vi "main.vi"(8 "error in":errorcluster) -> (0 "error out":errorcluster)   [LabVIEW 2018, in "Vehicle Position Interface.lvlib"]
uses:
  Vehicle Position Interface.lvlib
  Common/Common.lvlib
  Common/vi/Stop All - Action.ctl
  ctl/Queue Actions.ctl
  ctl/Module State.ctl
  Error Handler/Error Handler/ctl/Module State.ctl
  Error Handler/Error Handler/Error Handler.lvlib
  Controller/Controller.lvlib
  Controller/ctl/Module State.ctl
  ctl/Vehicle Position.ctl
panel:
  in  "Vehicle Position":T1 scale=0.0..4.0
  # "[Covers: UI1]"
  # "Vehicle Position Simulation"
  # "[Covers: UI4]"
  # "[Covers: UI4A]"
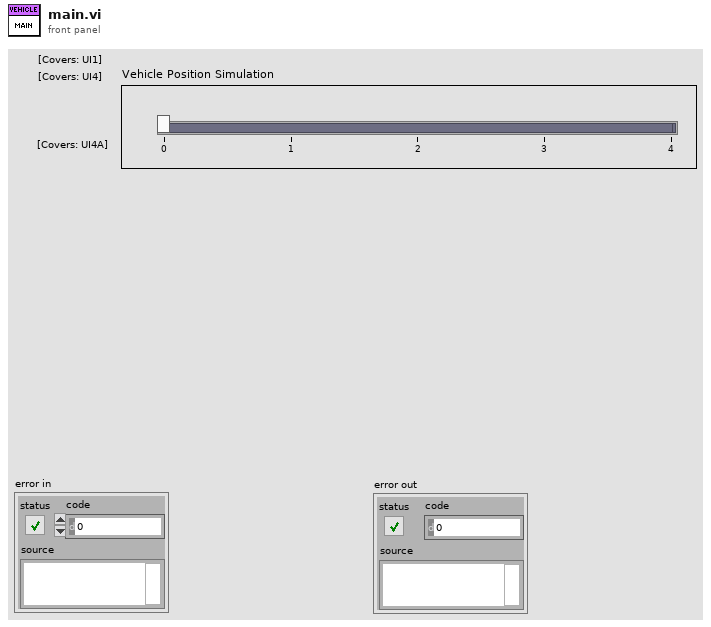
[diagram p1: front panel]
types:
  T1 = typedef "Vehicle Position Interface.lvlib/Vehicle Position.ctl" = dbl
  T2 = typedef "Vehicle Position Interface.lvlib/Module State.ctl" = enum16{"Init", "Idle", "Error", "Close", "Vehicle Position: Set", "Vehicle Position: Send to controller"}
  T3 = typedef "Vehicle Position Interface.lvlib/Queue Actions.ctl" = enum16{"Create", "Get", "Destroy"}
  T4 = typedef "Common.lvlib/Stop All - Action.ctl" = enum16{"Create", "Get", "Fire", "Destroy"}
  T5 = typedef "Controller.lvlib/Module State.ctl" = enum16{"Init", "Idle", "Error", "Close", "Wait for Start State", "Start State", "Wait For Vehicle Position", "Wash Step Execution", "Wash Step/Cycle Completion", "Wash Exit State", "Wash Abort/Terminate State", "Entry Console: Start button pressed", "Entry Console: Wash Steps buttons Pressed", "Vehicle Position: Slider Moved", "Check Timer"}
  T6 = typedef "Error Handler.lvlib/Module State.ctl" = enum16{"Init", "Idle", "Error", "Close", "Handle External Error", "Log Error"}
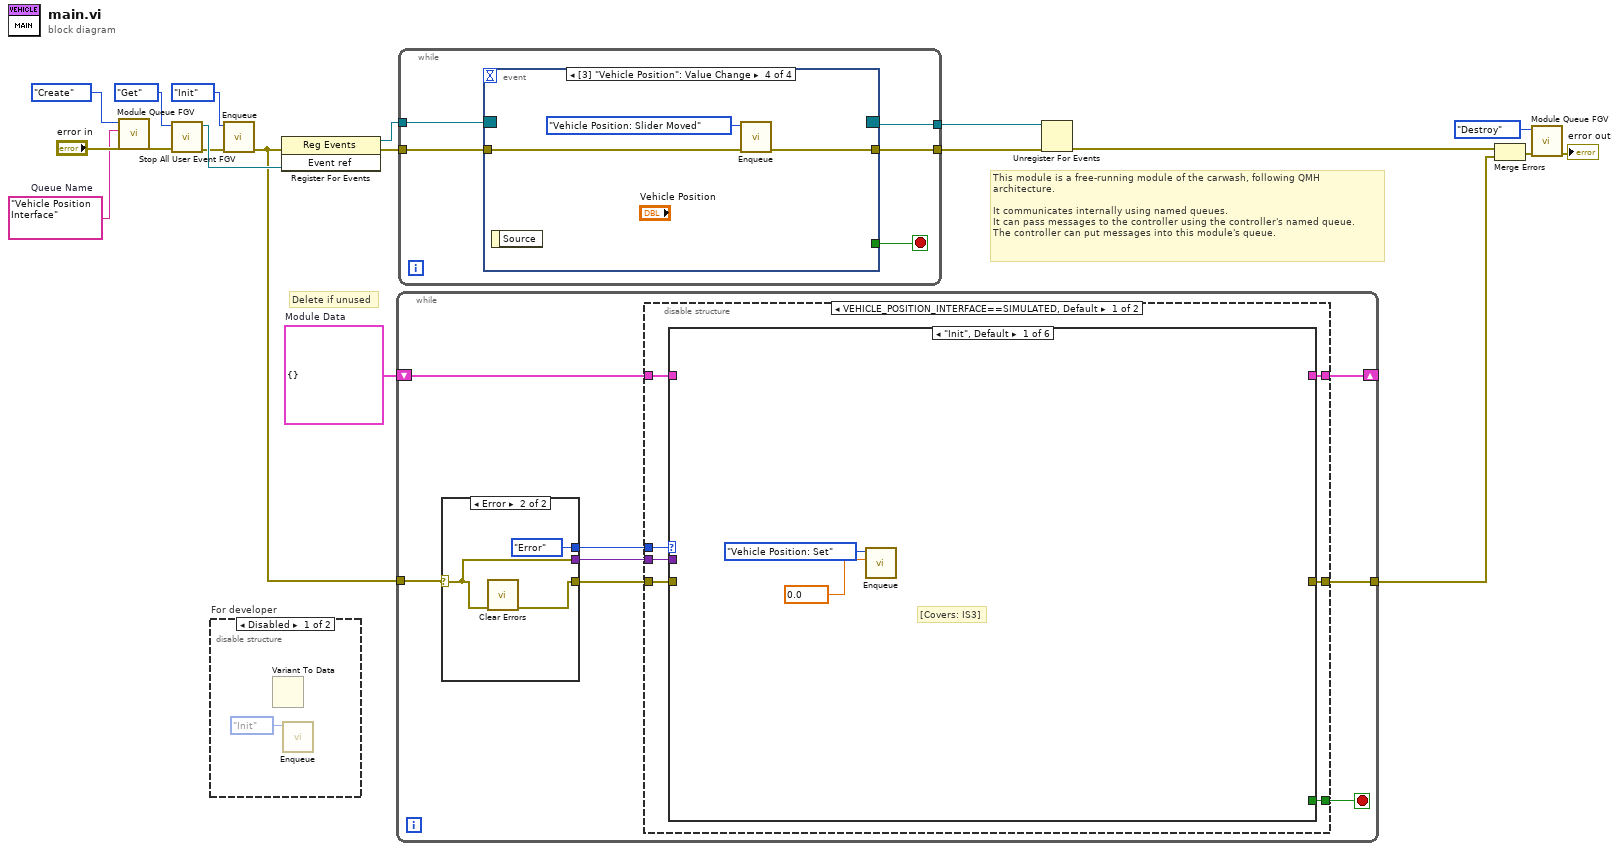
[diagram p0: block diagram]
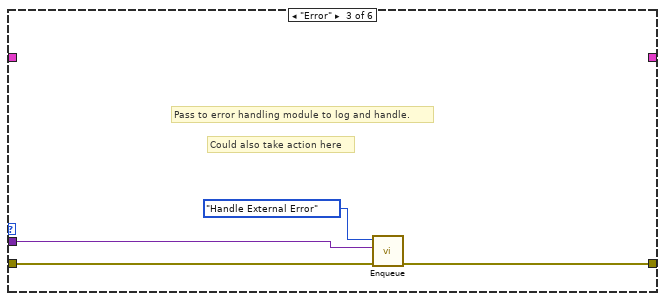
[diagram p4: hidden frame]
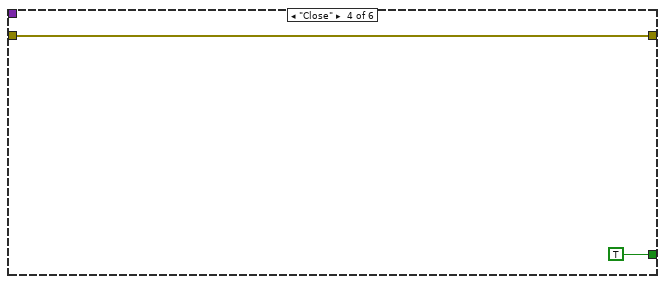
[diagram p5: hidden frame]
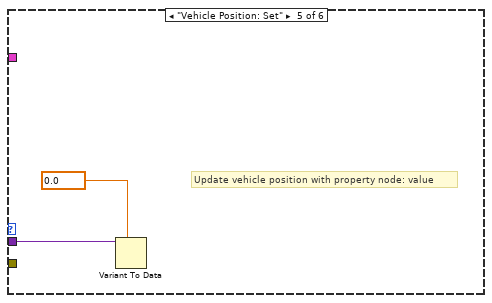
[diagram p6: hidden frame]
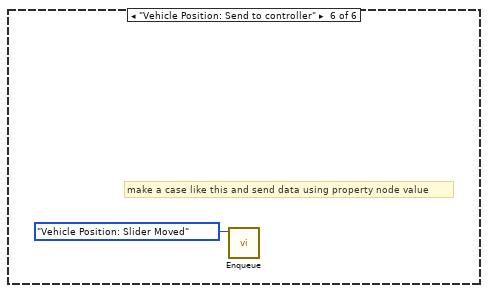
[diagram p7: hidden frame]
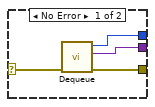
[diagram p9: hidden frame]
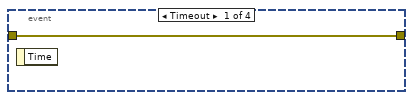
[diagram p10: hidden frame]
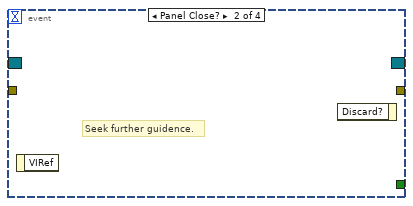
[diagram p11: hidden frame]
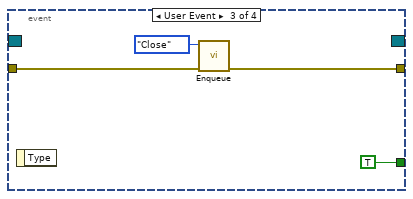
[diagram p12: hidden frame]
diagram:
  w1 = "Vehicle Position Interface"  # Queue Name
  w6 = cluster{} {}  # Module Data
  # "This module is a free-running module of the carwash, following QMH\narchitecture.\n\nIt communicates internally using named queues.\nIt can pass messages to the controller using the controller's named queue.\nThe controller can put messages into this module's queue."
  # "Delete if unused"
  n1 = call "Module Queue FGV.vi"("error in"="error in", "Queue Name"=w1, "Action"=Queue_Actions."Create") -> ("error out"=w16:errorcluster)  [unwired: 7 in, 1 out]
  n2 = call "Stop All User Event FGV.vi"("error in"=w16, "Action"=Stop_All_-_Action."Get") -> ("error out"=w15:errorcluster, "Event ref"=w18:refnum<user-event>)  [unwired: 8 in]
  n3 = disable-structure "For developer" shown="Disabled" {
    frame Disabled {
      n4 = Variant To Data() -> ()  [unwired: 3 in, 2 out]
      n5 = call "Enqueue.vi"("State"=Module_State."Init") -> ()  [unwired: 10 in, 1 out]
    }
    frame Enabled {
    }
  }
  n6 = call "Enqueue.vi"("error in"=w15, "State"=Module_State."Init") -> ("error out"=w7:errorcluster)  [unwired: 9 in]
  n7 = register-events(error in=w7, w18) -> (reference out=w13:refnum<event-registration>, error out=w11:errorcluster)  [unwired: 1 in]
  n8 = while {
    tunnel: w7 -> [w28]
    shift-right: [w23] -> _
    shift-left: w6 -> [w24]
    tunnel: [w21] -> w5
    stop <- w22 stop-if-true
    n9 = case shown="Error" w28 {
      selector: w28 -> [w51 w53]
      tunnel: [w50 w54] -> w25
      tunnel: [w49 w53] -> w26
      tunnel: [w48 Module_State."Error" ("State")] -> w27
      frame No Error {
        n10 = call "Dequeue.vi"("error in"=w51) -> ("error out"=w50:errorcluster, "Data"=w49:variant, "State"=w48:T2)  [unwired: 8 in]
      }
      frame Error {
        n11 = call <vilib>:"Clear Errors.vi"("error in (no error)"=w53) -> ("error out"=w54:errorcluster)  [unwired: 5 in, 1 out]
      }
    }
    n12 = disable-structure shown="VEHICLE_POSITION_INTERFACE==SIMULATED, Default" {
      disable-tunnel: w27 -> [w35 _]
      disable-tunnel: w26 -> [w34 _]
      disable-tunnel: w25 -> [w33 _]
      disable-tunnel: w24 -> [w32 _]
      disable-tunnel: [w31 _] -> w23
      disable-tunnel: [w30 _] -> w22
      disable-tunnel: [w29 _] -> w21
      frame condition #0 (active) {
        n13 = case shown="\"Init\", Default" w35 {
          tunnel: w34 -> [_ _ w40 _ w45 _]
          tunnel: w33 -> [_ _ w39 w43 _ _]
          tunnel: w32 -> [_ w38 _ _ _ _]
          tunnel: [_ w38 _ _ _ _] -> w31
          tunnel: [_ _ _ TRUE _ _] -> w30
          tunnel: [_ _ w41 w43 _ _] -> w29
          frame "Init", Default {
            w36 = 0.0 items=["Entry", "Station 1", "Station 2", "Station 3", "Exit"] ("Vehicle Position")
            # "[Covers: IS3]"
            n14 = call "Enqueue.vi"("Data"=w36, "State"=Module_State."Vehicle Position: Set") -> ()  [unwired: 9 in, 1 out]
          }
          frame "Idle" {
          }
          frame "Error" {
            # "Could also take action here"
            # "Pass to error handling module to log and handle."
            n15 = call "Enqueue.vi"("error in"=w39, "Data"=w40, "State"=Module_State."Handle External Error") -> ("error out"=w41:errorcluster)  [unwired: 8 in]
          }
          frame "Close" {
          }
          frame "Vehicle Position: Set" {
            w46 = 0.0 items=["Entry", "Station 1", "Station 2", "Station 3", "Exit"] ("Vehicle Position")
            # "Update vehicle position with property node: value"
            n16 = Variant To Data(type=w46, Variant=w45) -> ()  [unwired: 1 in, 2 out]
          }
          frame "Vehicle Position: Send to controller" {
            # "make a case like this and send data using property node value"
            n17 = call "Enqueue.vi"("State"=Module_State."Vehicle Position: Slider Moved") -> ()  [unwired: 10 in, 1 out]
          }
        }
      }
      frame condition #1 {
      }
    }
  }
  n18 = while {
    tunnel: w13 -> [w59]
    tunnel: [w58] -> w12
    tunnel: [w57] -> w10
    tunnel: w11 -> [w56]
    stop <- w55 stop-if-true
    n19 = event shown="[3] \"Vehicle Position\": Value Change" {
      selector: w59 -> [_ _ _ _]
      dyn-events: [_ _ _ _] -> w58
      timeout: _ -> [_ _ _ _]
      tunnel: [w60 _ w63 w65] -> w57
      tunnel: w56 -> [w60 _ w64 w66]
      tunnel: [_ _ TRUE _] -> w55
      event Timeout {
        n20 = event-data() -> ()  [unwired: 1 in, 1 out]
      }
      event Panel Close? {
        # "Seek further guidence."
        n21 = event-data() -> ()  [unwired: 1 in, 1 out]
        n22 = event-data() -> ()  [unwired: 2 in, 1 out]
      }
      event User Event {
        n23 = event-data() -> ()  [unwired: 1 in, 1 out]
        n24 = call "Enqueue.vi"("error in"=w64, "State"=Module_State."Close") -> ("error out"=w63:errorcluster)  [unwired: 9 in]
      }
      event Value Change {
        n25 = event-data() -> ()  [unwired: 1 in, 1 out]
        n26 = call "Enqueue.vi"("error in"=w66, "State"=Module_State."Vehicle Position: Slider Moved") -> ("error out"=w65:errorcluster)  [unwired: 9 in]
      }
    }
  }
  n27 = Unregister For Events(event registration refnum=w12, error in=w10) -> (error out=w2:errorcluster)
  n28 = Merge Errors(w2, w5) -> (w4:errorcluster)
  n29 = call "Module Queue FGV.vi"("error in"=w4, "Action"=Queue_Actions."Destroy") -> ("error out"=→"error out":errorcluster)  [unwired: 8 in, 1 out]
